vi "StellarNet Initialize Operating Parameters.vi"(8 "error in":errorcluster, 9 "Spectrometer Coefficients file":path=path "StellarNet Spectrometer Coefficients.xml", 10 "Location of SpectraWiz":path=path "C:/program files/StellarNet/SpectraWiz", 11 "Number of Channels":i32) -> (0 "error out":errorcluster, 2 "Operating Parameters":T1(array[cluster]) {"Digitizer Clock Rate Setting" min=1 max=3; "Optical Smoothing Level" min=0 max=4 step=1; "Number of Scans to Average" min=1 max=10000 step=1})   [LabVIEW 2023]
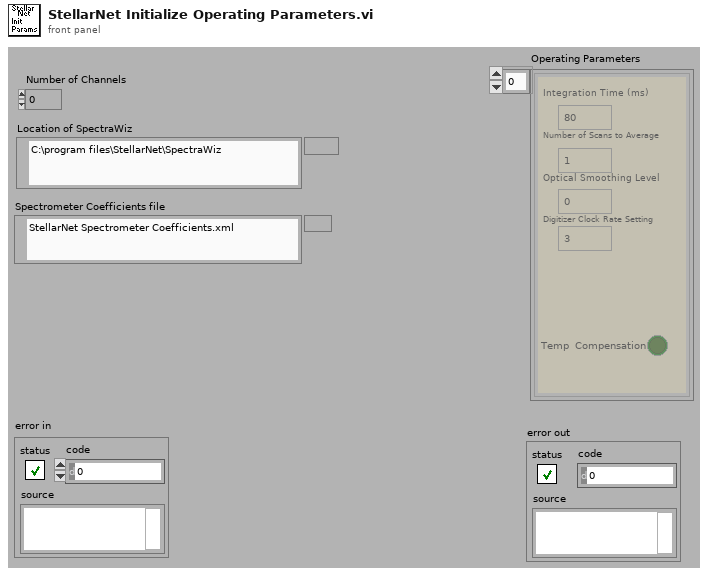
[diagram p1: front panel]
types:
  T1 = cluster{"Integration Time (ms)":i32, "Number of Scans to Average":i32, "Optical Smoothing Level":i32, "Digitizer Clock Rate Setting":i32, "Temp  Compensation ":bool}[]
  T2 = cluster{"Integration Time (ms)":i32, "Number of Scans to Average":i32, "Optical Smoothing Level":i32, "Digitizer Clock Rate Setting":i32, "Temp  Compensation":bool}
  T3 = cluster{"Integration Time (ms)":i32, "Number of Scans to Average":i32, "Optical Smoothing Level":i32, "Digitizer Clock Rate Setting":i32, "Drift Correct":bool}[]
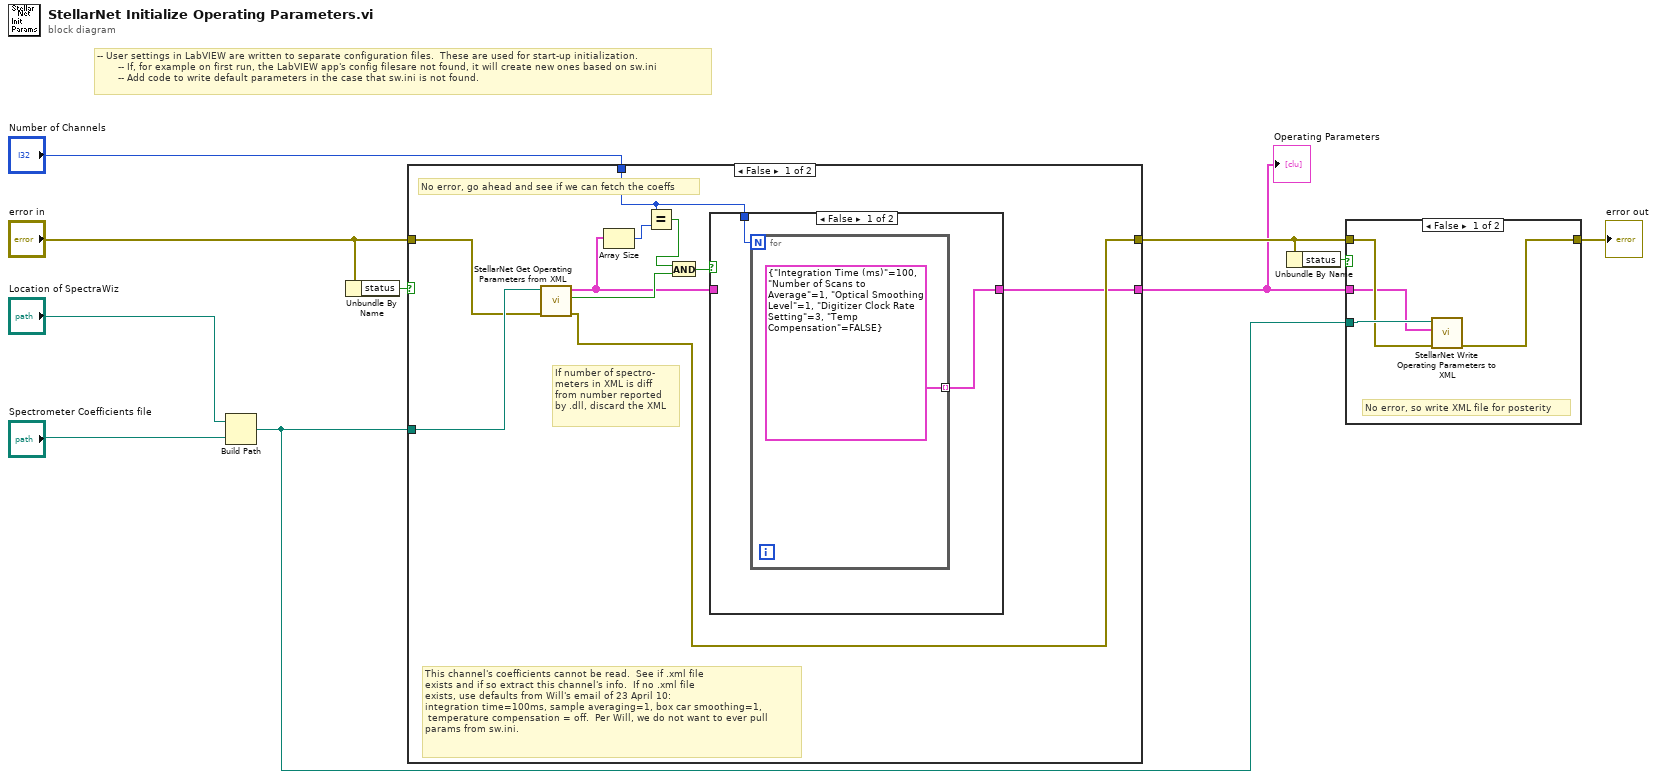
[diagram p0: block diagram]
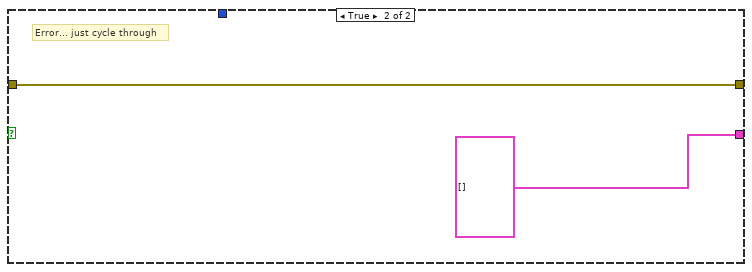
[diagram p3: hidden frame]
diagram:
  # "-- User settings in LabVIEW are written to separate configuration files.  These are used for start-up initialization.\n       -- If, for example on first run, the LabVIEW app's config filesare not found, it will create new ones based on sw.ini\n       -- Add code to write default parameters in the case that sw.ini is not found."
  n1 = Build Path(base path="Location of SpectraWiz", name or relative path="Spectrometer Coefficients file") -> (appended path=w5:path)
  n2 = Unbundle By Name("error in") -> ("status"=w2:bool)
  n3 = case shown="False" w2 {
    tunnel: "error in" -> [w19 w26]
    tunnel: [w14 w26] -> w7
    tunnel: w5 -> [w20 _]
    tunnel: "Number of Channels" -> [w13 _]
    tunnel: [w12 T3 [] ("Operating Parameters")] -> w1
    frame False {
      # "If number of spectro-\nmeters in XML is diff\nfrom number reported\nby .dll, discard the XML"
      # "This channel's coefficients cannot be read.  See if .xml file \nexists and if so extract this channel's info.  If no .xml file \nexists, use defaults from Will's email of 23 April 10:\nintegration time=100ms, sample averaging=1, box car smoothing=1,\n temperature compensation = off.  Per Will, we do not want to ever pull\nparams from sw.ini."
      # "No error, go ahead and see if we can fetch the coeffs"
      n4 = call "StellarNet Get Operating Parameters from XML.vi"("error in (no error)"=w19, "XML File Path"=w20) -> ("error out"=w14:errorcluster, "file or folder exists?"=w16:bool, "Operating Parameters"=w11:T1)  [unwired: 7 in]
      n5 = Array Size(array=w11) -> (size(s)=w18:i32)
      n6 = Equal?(x=w13, y=w18) -> (x = y?=w17:bool)
      n7 = And(x=w17, y=w16) -> (x .and. y?=w15:bool)
      n8 = case shown="False" w15 {
        tunnel: w13 -> [w22 _]
        tunnel: w11 -> [_ w24]
        tunnel: [w21 w24] -> w12
        frame False {
          n9 = for {
            N: w22 -> [_]
            tunnel: [T2 {"Integration Time (ms)"=100, "Number of Scans to Average"=1, "Optical Smoothing Level"=1, "Digitizer Clock Rate Setting"=3, "Temp  Compensation"=FALSE} ("Operation Settings")] -> w21 mode=indexing
          }
        }
        frame True {
        }
      }
    }
    frame True {
      # "Error... just cycle through"
    }
  }
  "Operating Parameters" <- w1
  n10 = Unbundle By Name(w7) -> ("status"=w8:bool)
  n11 = case shown="False" w8 {
    tunnel: w7 -> [w29 w31]
    tunnel: [w28 w31] -> w6
    tunnel: w5 -> [w30 _]
    tunnel: w1 -> [w27 _]
    frame False {
      # "No error, so write XML file for posterity"
      n12 = call "StellarNet Write Operating Parameters to XML.vi"("error in (no error)"=w29, "Operating Parameters"=w27, "XML File Path"=w30) -> ("error out"=w28:errorcluster)  [unwired: 8 in]
    }
    frame True {
    }
  }
  "error out" <- w6
